vi "Tester.vi"() -> ()   [LabVIEW 2014, in "CAP-USB-1.lvlib"]
uses:
  CAP-USB-1.lvlib
  CAP-USB-1Class/CAP-USB-1.lvclass
panel:
  out "Acquisition Data":cluster{"TDX":sgl[], "TDX Index":u32[]}[](array[cluster])
  in  "stop":bool
  out "Control Data":T1
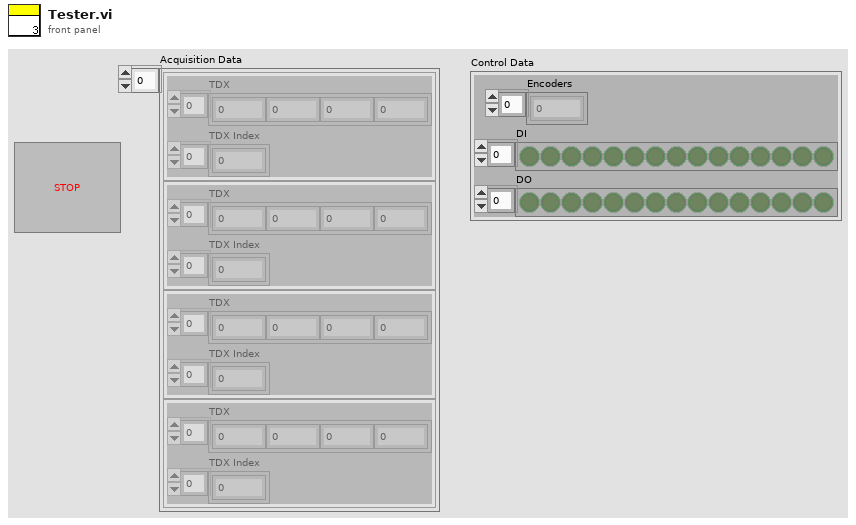
[diagram p1: front panel]
types:
  T1 = cluster{"Encoders":i32[], "DI":bool[], "DO":bool[]}
  T2 = typedef "DriverMasterSync.lvlibp/WINFAS 2 Data Queue.lvlib/Control Data Cluster.ctl" = cluster{"Encoder":sgl, "DI":bool[], "DO":bool[]}
  T3 = typedef "DriverMasterSync.lvlibp/WINFAS 2 Data Queue.lvlib/Acquisition Data Cluster.ctl" = T4[]
  T4 = typedef "DriverMasterSync.lvlibp/WINFAS 2 Data Queue.lvlib/Acquisition Data 1 Sample Cluster.ctl" = cluster{"TDX":sgl[], "Encoder":sgl}
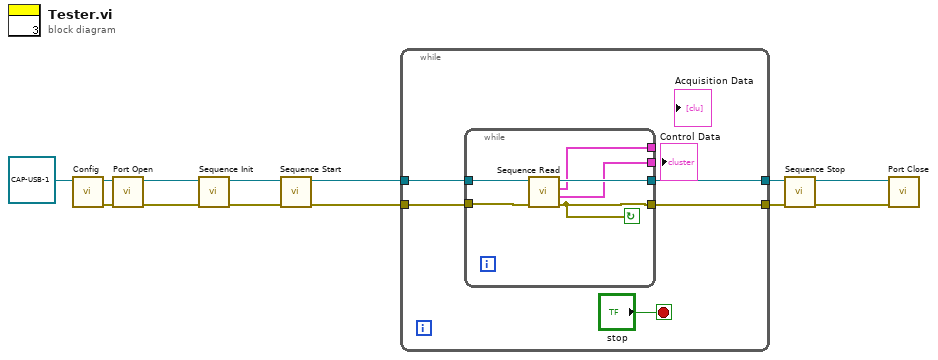
[diagram p0: block diagram]
diagram:
  n1 = call-dynamic "Config.vi"("CAP-USB-1 in"=refnum<class "CAP-USB-1.lvclass"> refnum) -> ("error out"=w9:errorcluster, "CAP-USB-1 out"=w13:refnum<class "CAP-USB-1.lvclass">)  [unwired: 8 in, 1 out]
  n2 = call-dynamic "Port Open.vi"("error in (no error)"=w9, "CAP-USB-1 in"=w13) -> ("error out"=w8:errorcluster, "CAP-USB-1 out"=w12:refnum<class "CAP-USB-1.lvclass">)  [unwired: 8 in]
  n3 = call-dynamic "Sequence Init.vi"("error in (no error)"=w8, "CAP-USB-1 in"=w12) -> ("error out"=w7:errorcluster, "CAP-USB-1 out"=w11:refnum<class "CAP-USB-1.lvclass">)  [unwired: 8 in]
  n4 = call-dynamic "Sequence Start.vi"("error in (no error)"=w7, "CAP-USB-1 in"=w11) -> ("error out"=w6:errorcluster, "CAP-USB-1 out"=w10:refnum<class "CAP-USB-1.lvclass">)  [unwired: 8 in]
  n5 = while {
    tunnel: w6 -> [w17]
    tunnel: [w15] -> w4
    tunnel: w10 -> [w18]
    tunnel: [w16] -> w5
    stop <- "stop" stop-if-true
    n6 = while {
      tunnel: w18 -> [w24]
      tunnel: w17 -> [w23]
      tunnel: [w22] -> w16
      tunnel: [w21] -> w15
      tunnel: [w20] -> _
      tunnel: [w19] -> _
      stop <- w21 continue-if-true
      n7 = call-dynamic "Sequence Read.vi"("error in (no error)"=w23, "CAP-USB-1 in"=w24) -> ("error out"=w21:errorcluster, "Control Data"=w19:T2, "Acquisition Data"=w20:T3, "CAP-USB-1 out"=w22:refnum<class "CAP-USB-1.lvclass">)  [unwired: 6 in]
    }
  }
  n8 = call-dynamic "Sequence Stop.vi"("error in (no error)"=w4, "CAP-USB-1 in"=w5) -> ("error out"=w2:errorcluster, "CAP-USB-1 out"=w3:refnum<class "CAP-USB-1.lvclass">)  [unwired: 8 in]
  n9 = call-dynamic "Port Close.vi"("error in (no error)"=w2, "CAP-USB-1 in"=w3) -> ()  [unwired: 8 in, 2 out]
